vi "PulseClosing.vi"(6 "Reset Relay":bool, 8 "Pulse Index In":i32, 9 "State In":T1(ring)=enum."Wait for Trip", 10 "Trip signal":bool, 11 "Time lapsed":u32) -> (0 "Pulse Index Out":i32, 1 "State Out":T1(ring)=enum."Wait for Trip", 2 "Reclose":bool)   [LabVIEW 2016]
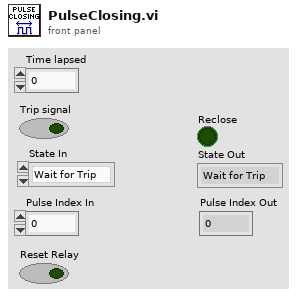
[diagram p1: front panel]
types:
  T1 = enum16{"Idle", "Wait for Trip", "PulseClosing", "Locked"}
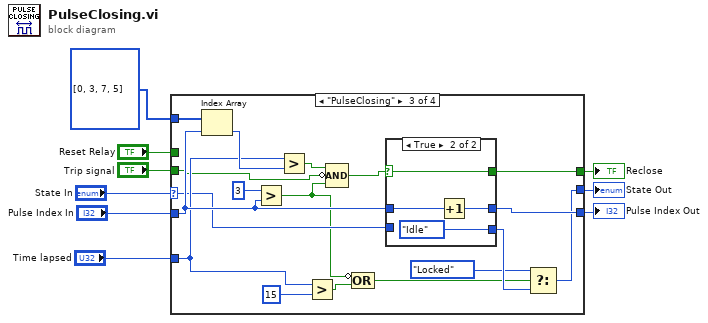
[diagram p0: block diagram]
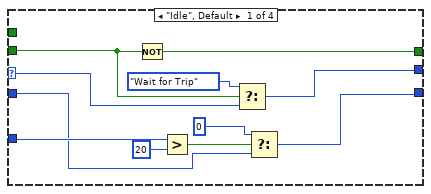
[diagram p2: hidden frame]
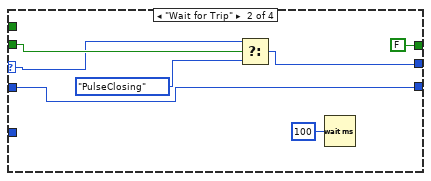
[diagram p3: hidden frame]
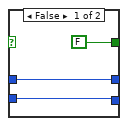
[diagram p4: hidden frame]
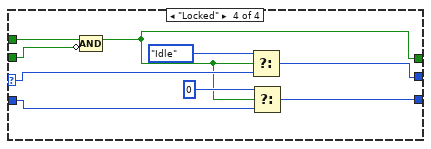
[diagram p5: hidden frame]
diagram:
  n1 = case shown="\"PulseClosing\"" "State In" {
    selector: "State In" -> [w20 w26 w32 w60]
    tunnel: [w16 FALSE w42 w54] -> w9
    tunnel: "Trip signal" -> [w17 w27 w33 w56]
    tunnel: [w18 w24 w36 w58] -> w1
    tunnel: "Pulse Index In" -> [w12 w22 w39 w61]
    tunnel: "Reset Relay" -> [_ _ _ w57]
    tunnel: u32[] [0, 3, 7, 5] -> [_ _ w41 _]
    tunnel: [w10 w22 w40 w55] -> w4
    tunnel: "Time lapsed" -> [w15 _ w37 _]
    frame "Idle", Default {
      n2 = Not(x=w17) -> (.not. x?=w16:bool)
      n3 = Greater?(x=w15, y=u32 20) -> (0:w13:bool)
      n4 = Select(t=T1."Wait for Trip", s=w17, f=w20) -> (s? t:f=w18:T1)
      n5 = Select(t=0 ("y"), s=w13, f=w12) -> (s? t:f=w10:i32)
    }
    frame "Wait for Trip" {
      n6 = Select(t=w26, s=w27, f=T1."PulseClosing") -> (s? t:f=w24:T1)
      n7 = Wait (ms)(milliseconds to wait=u32 100) -> ()  [unwired: 1 out]
    }
    frame "PulseClosing" {
      n8 = Index Array(array=w41, index=w39) -> (element=w38:u32)
      n9 = Greater?(x=3, y=w39) -> (0:w30:bool)
      n10 = Greater?(x=w37, y=w38) -> (0:w44:bool)
      n11 = Greater?(x=w37, y=u32 15) -> (0:w34:bool)
      n12 = Compound Arithmetic op=AND(w44, invert w33, w30) -> (w43:bool)
      n13 = Compound Arithmetic op=OR(invert w30, w34) -> (w29:bool)
      n14 = case shown="True" w43 {
        selector: w43 -> [_ w52]
        tunnel: [FALSE w52] -> w42
        tunnel: [w47 w51] -> w40
        tunnel: w39 -> [w47 w50]
        tunnel: [w46 T1."Idle"] -> w31
        tunnel: w32 -> [w46 _]
        frame False {
        }
        frame True {
          n15 = Increment(x=w50) -> (x+1=w51:i32)
        }
      }
      n16 = Select(t=T1."Locked", s=w29, f=w31) -> (s? t:f=w36:T1)
    }
    frame "Locked" {
      n17 = Compound Arithmetic op=AND(w57, invert w56) -> (w54:bool)
      n18 = Select(t=T1."Idle", s=w54, f=w60) -> (s? t:f=w58:T1)
      n19 = Select(t=0 ("Pulse Index In"), s=w54, f=w61) -> (s? t:f=w55:i32)
    }
  }
  "Reclose" <- w9
  "Pulse Index Out" <- w4
  "State Out" <- w1
